vi "DataLogViewer.vi"() -> ()   [LabVIEW 2017]
uses:
  <vilib>/Utility/miscctls.llb/LVRowAndColumnTypeDef.ctl
  <vilib>/Utility/miscctls.llb/LVRowAndColumnUnsignedTypeDef.ctl
  <vilib>/Utility/sysdir.llb/System Directory Type.ctl
  <vilib>/Utility/NIReport.llb/Append Image to Report (path wrap).vi
  <vilib>/Utility/file.llb/Read Delimited Spreadsheet (string).vi
  <vilib>/Utility/NIReport.llb/NI_report.lvclass
  <vilib>/Utility/NIReport.llb/NI_ReportGenerationCore.lvlib
panel:
  in  "Print":bool
  in  "Explorer":bool
  out "SearchOut":T1
  in  "Search":bool
  in  "STR_Search":string caption="Search..."
  in  "Down":bool
  in  "Top":bool
  out "ResultGraph":string[](array[string])
  out "ResultTest":string[][](array[string])
  in  "Tab Control":enum32{"RESULT", "GRAPH"}(tab)
  out "PRODUCT No.":string
  out "LANE  No.":string
  out "LASER  No.":string
  out "RESULT":string
  out "QR Code":string
  out "Vision Pin":string
  out "Vision Pad":string
  out "LIN WDW Lock":string
  out "LIN AS Auto":string
  out "LIN AS Down":string
  out "LIN AS Up":string
  out "LIN DR Auto":string
  out "LIN DR Down":string
  out "LIN DR Up":string
  out "RL Man Down":string
  out "RL Man Up":string
  out "FL Auto Down":string
  out "FL Auto Up":string
  out "FL Man Down":string
  out "FL Man Up":string
  out "RR Man Down":string
  out "RR Man Up":string
  out "FR Auto Down":string
  out "FR Auto Up":string
  out "FR Man Down":string
  out "FR Man Up":string
  out "Door Unlocked":string
  out "Door Lock":string
  out "WDW Unlocked":string
  out "WDW Locked":string
  out "Megga Test":string
  out "RLG_Up":picture
  out "RLG_Down":picture
  out "FLG_Up":picture
  out "FLG_Down":picture
  out "RRG_Up":picture
  out "RRG_Down":picture
  out "FRG_Up":picture
  out "FRG_Down":picture
  out "DLG_Unlock":picture
  out "DLG_Lock":picture
  out "WDWG_Unlock":picture
  out "WDWG_Lock":picture
  out "FileCount":string
  out "Display":bool
  in  "TableType":string(combo)="VIEW ALL"
  out "Folder Table":string[][](table)
  in  "RefreshFolderList":bool
  out "DataC4":string[](array[string])
  out "PathC3":path
  out "PathC2":path
  out "DataC3":string[](array[string])
  out "DataC2":string[](array[string])
  out "DataC1":string[](array[string])
  out "PathC1":path
  out "PosC3":T2
  out "PosC2":T2
  in  "MasterPath":path=path "D:/Output"
  out "PosC1":T2
  # "RL Down"
  # "RL Up"
  # "FL Down"
  # "FL Up"
  # "RR Down"
  # "RR Up"
  # "FR Down"
  # "FR Up"
  # "Door Lock"
  # "Door Unlock"
  # "WDW Lock"
  # "WDW Unlock"
  # "DATA LOGGER"
  # "DATA LOGGER"
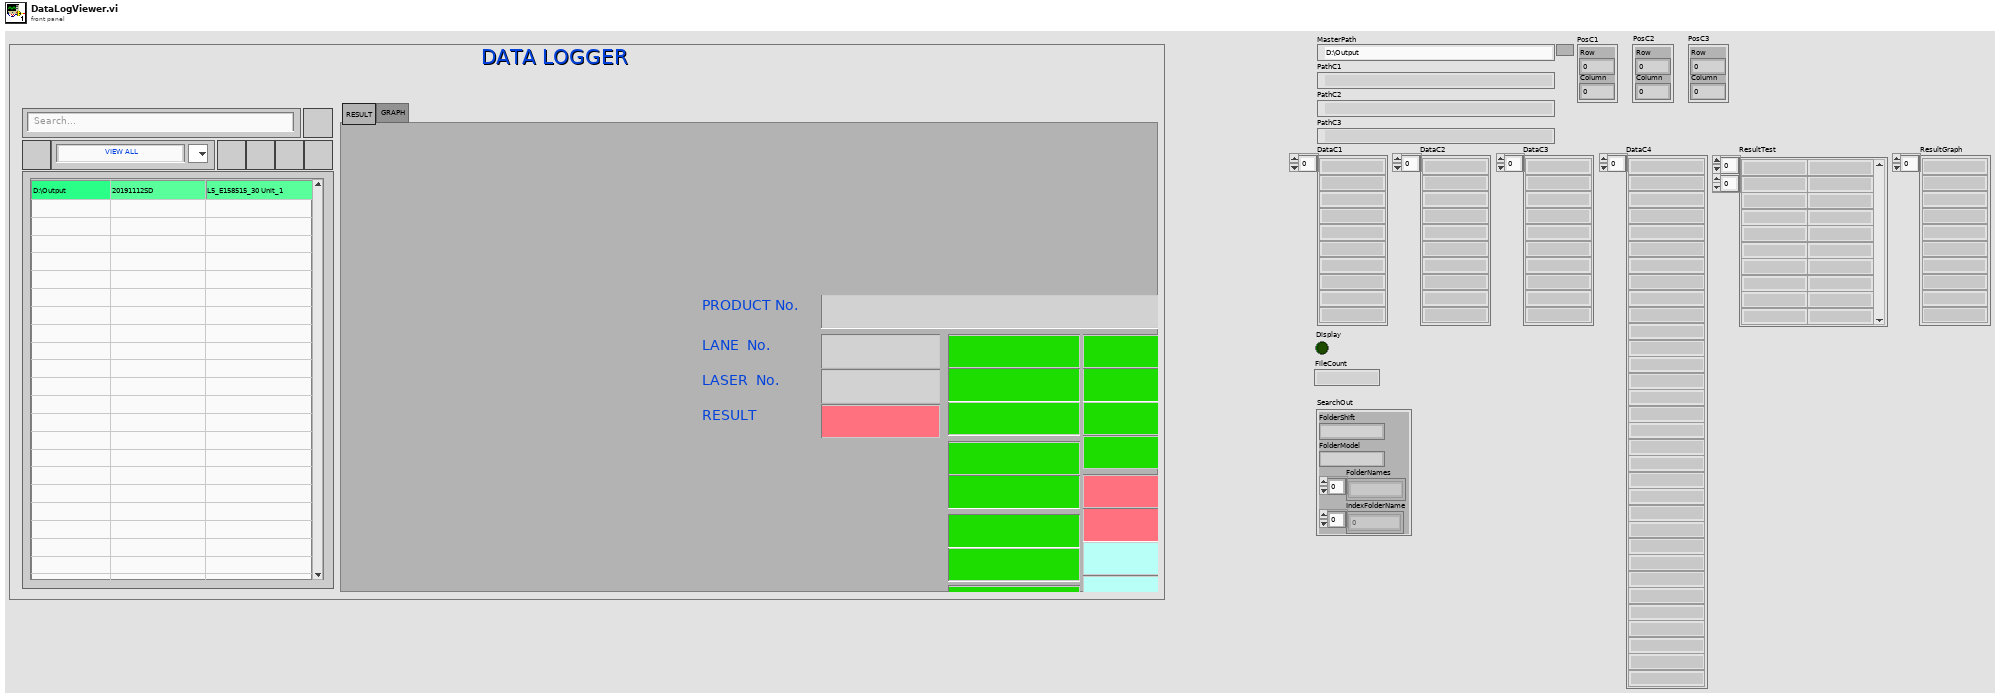
[diagram p1: front panel]
types:
  T1 = cluster{"FolderShift":string, "FolderModel":string, "FolderNames":string[], "IndexFolderName":i32[]}
  T2 = typedef "LVRowAndColumnTypeDef.ctl" = cluster{"Row":i32, "Column":i32}
  T3 = typedef "LVRowAndColumnUnsignedTypeDef.ctl" = cluster{"Row":u32, "Column":u32}
  T4 = enum16{"Standard Report", "HTML", "Word", "Excel"}
  T5 = enum16{"maximized", "minimized", "normal", "no change"}
  T6 = cluster{"top":dbl, "left":dbl, "right":dbl, "bottom":dbl}
  T7 = typedef "System Directory Type.ctl" = i32
  T8 = typedef "imagedata.ctl" = cluster{"image type":i32, "image depth":i32, "image":u8[], "mask":u8[], "colors":u32[], "Rectangle":cluster{"left":i16, "top":i16, "right":i16, "bottom":i16}}
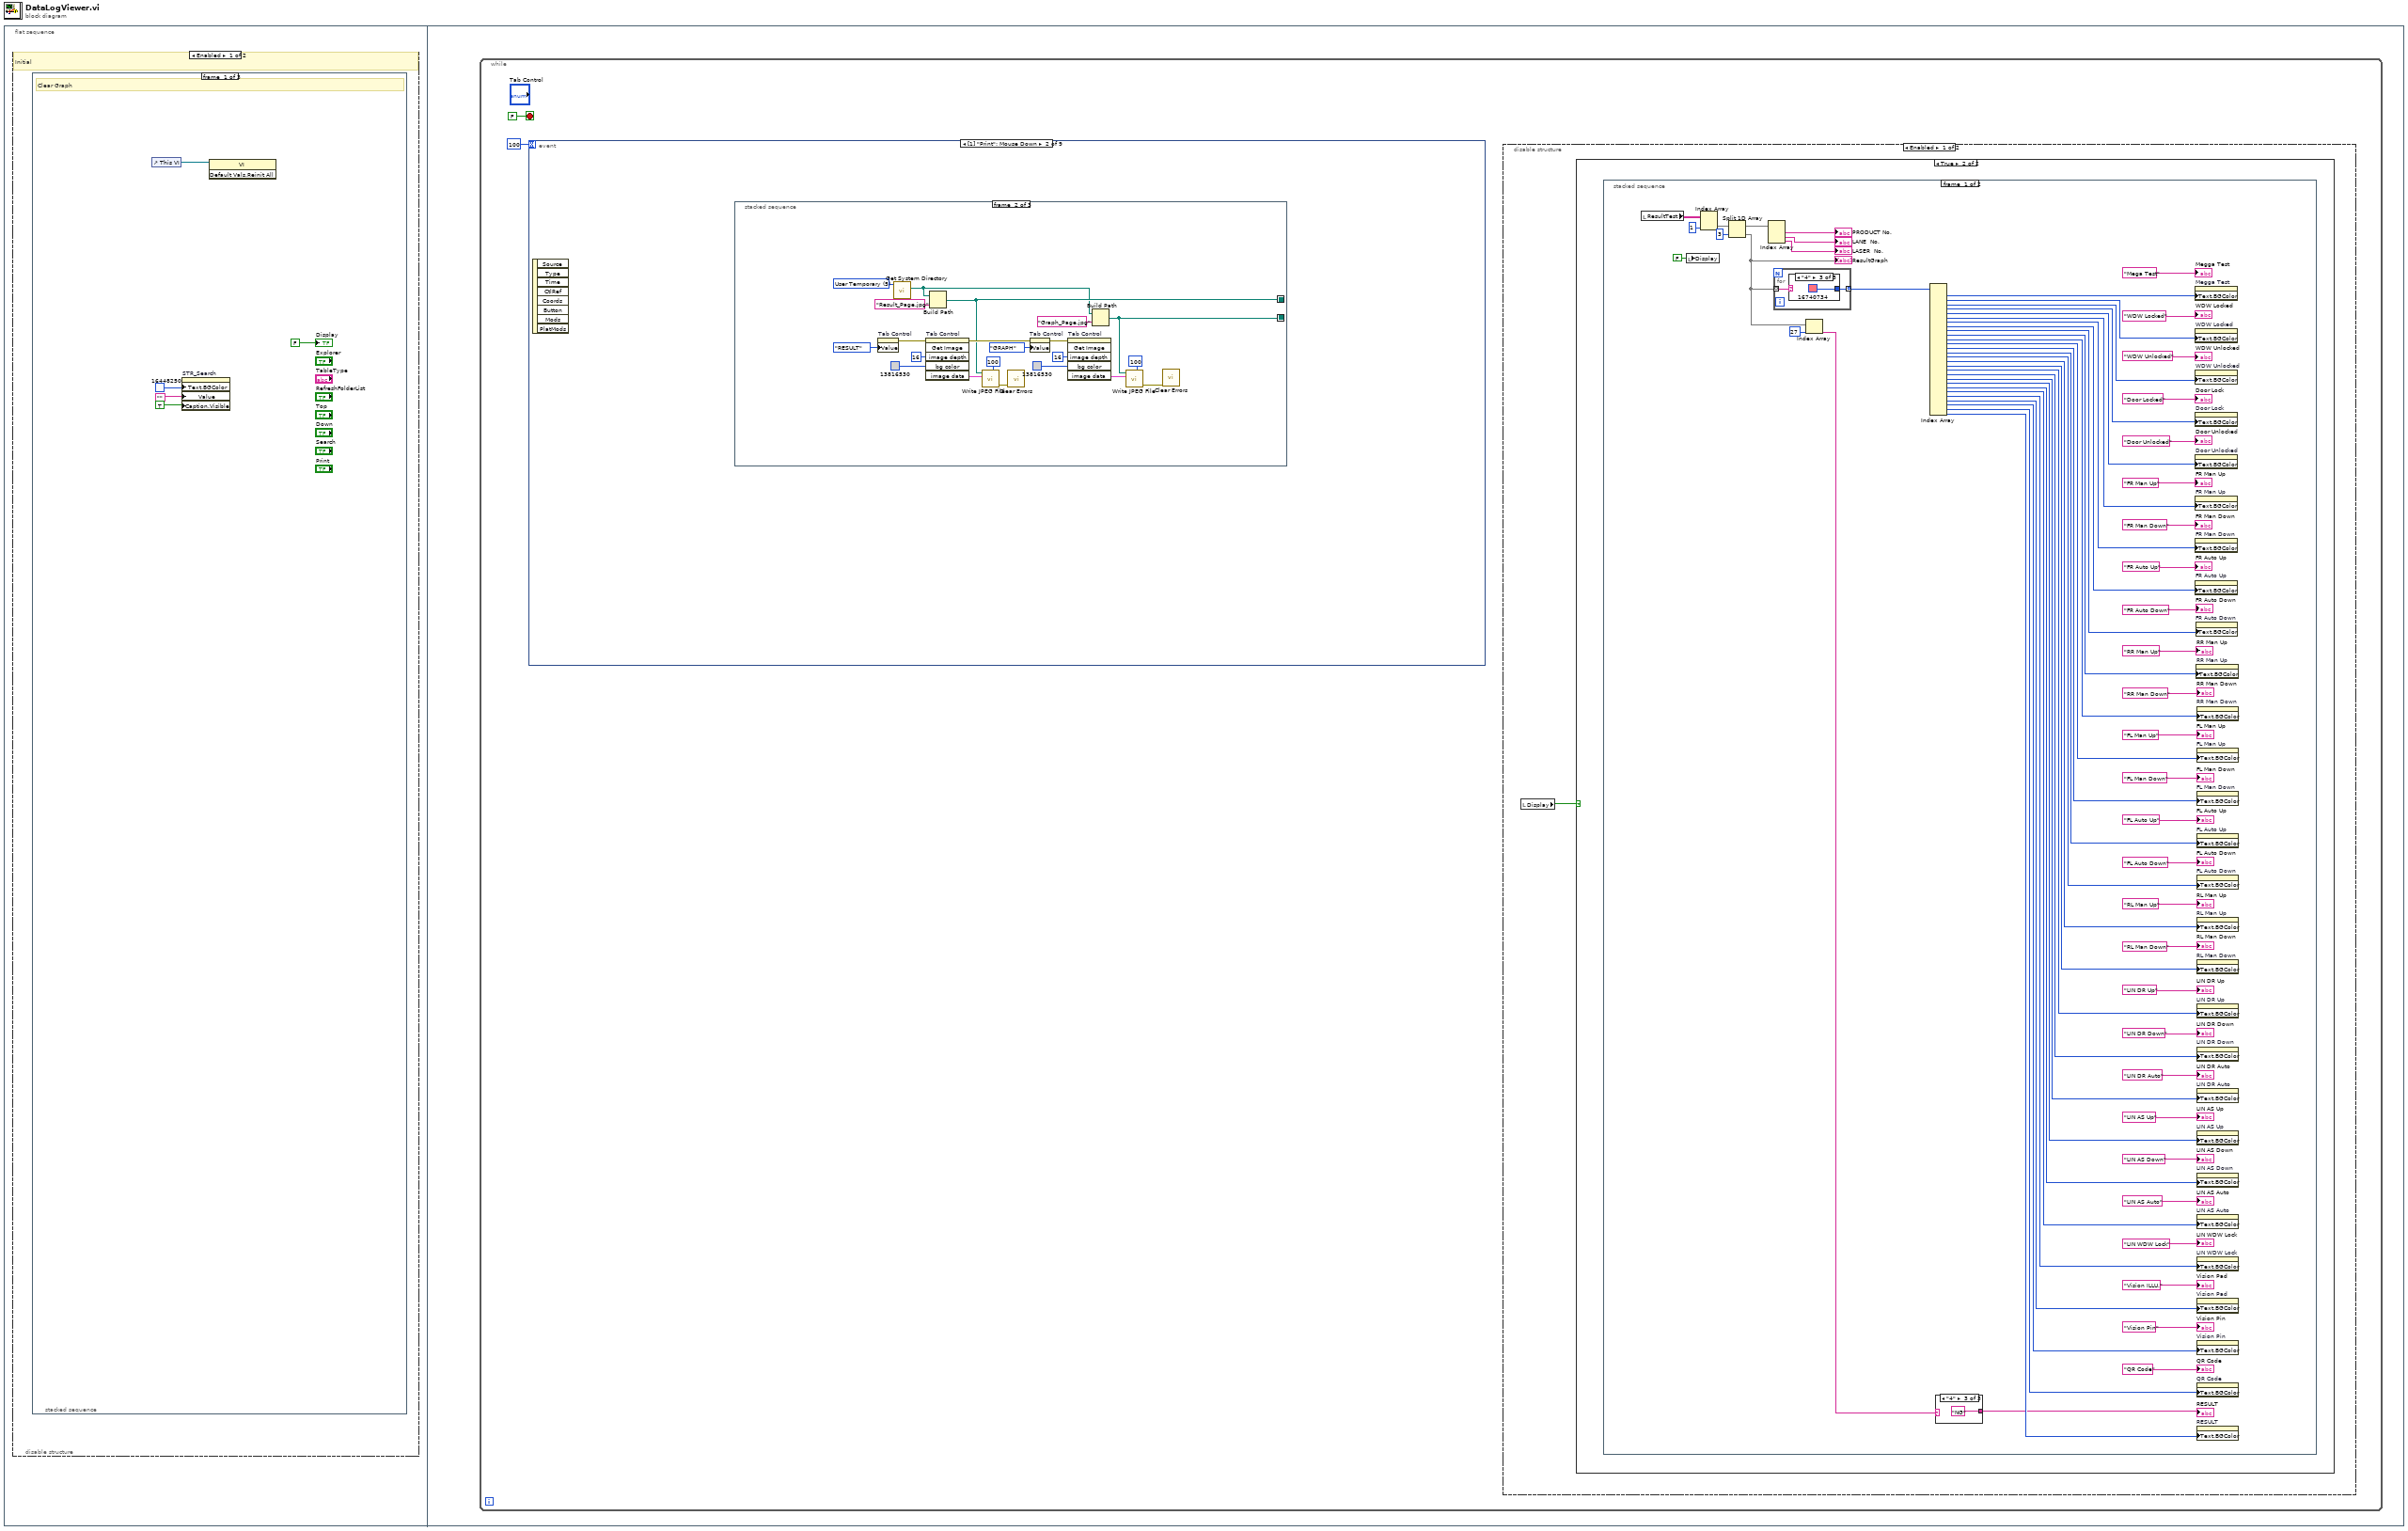
[diagram p0: block diagram]
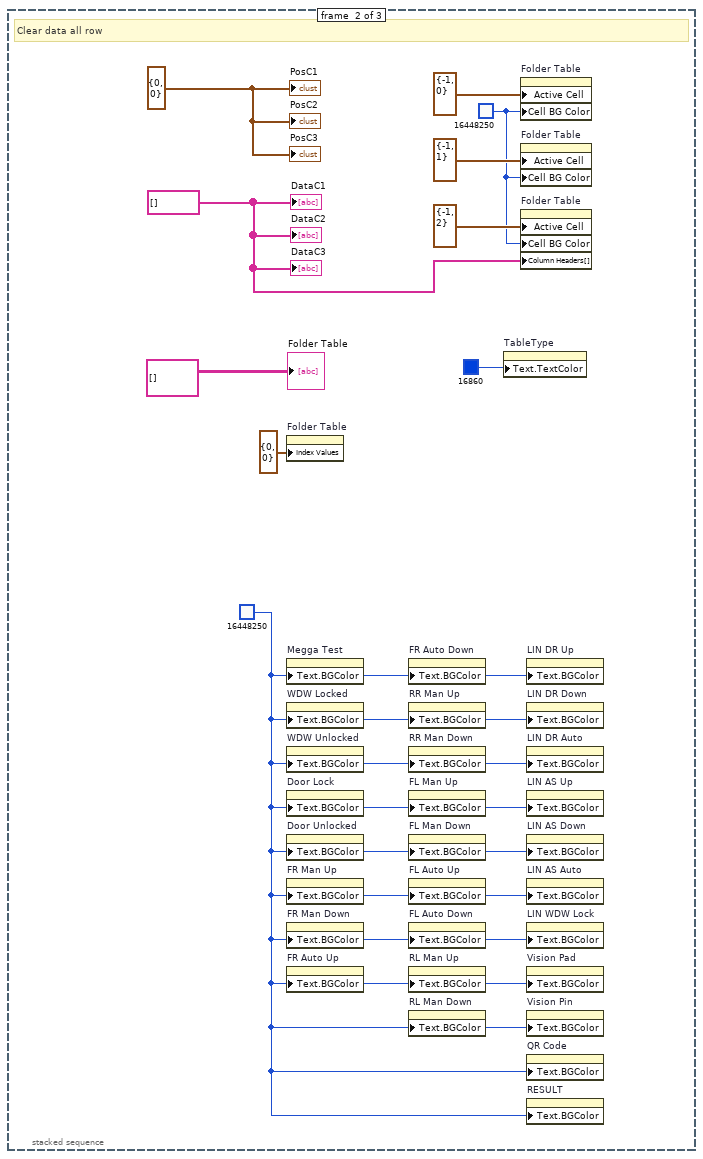
[diagram p2: hidden frame]
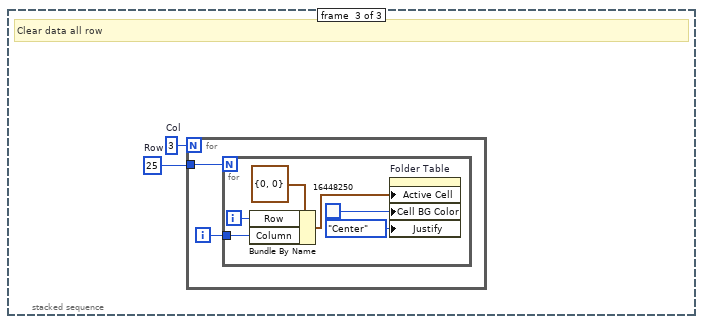
[diagram p3: hidden frame]
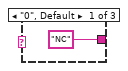
[diagram p6: hidden frame]
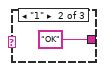
[diagram p7: hidden frame]
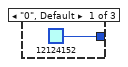
[diagram p8: hidden frame]
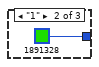
[diagram p9: hidden frame]
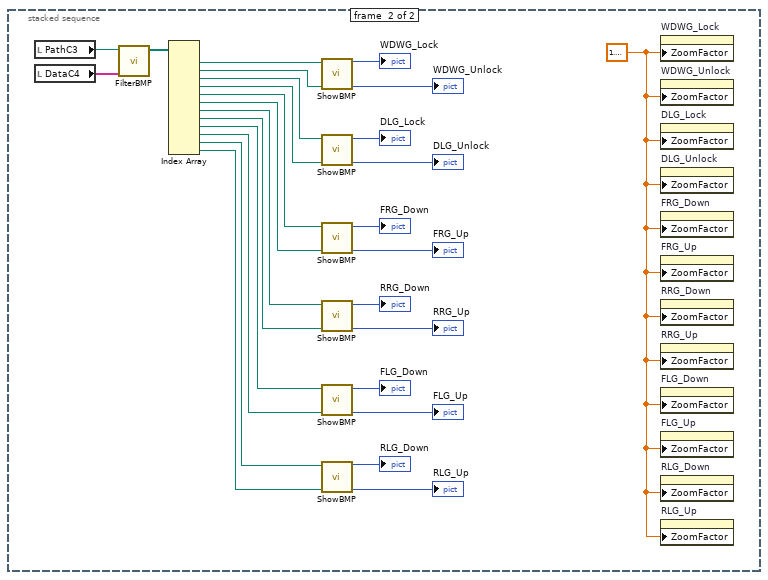
[diagram p10: hidden frame]
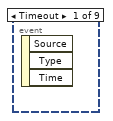
[diagram p12: hidden frame]
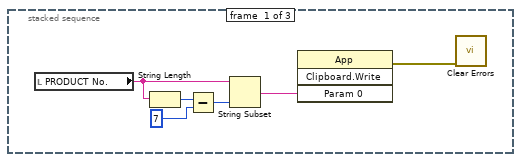
[diagram p13: hidden frame]
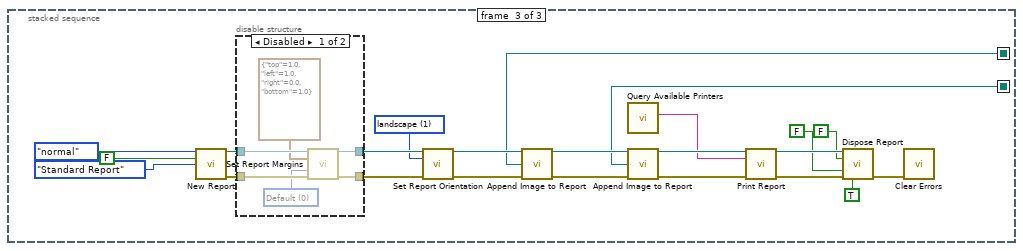
[diagram p14: hidden frame]
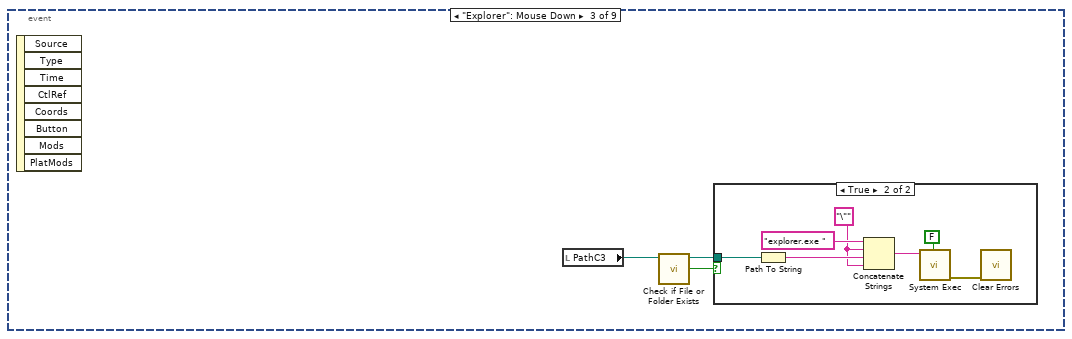
[diagram p16: hidden frame]
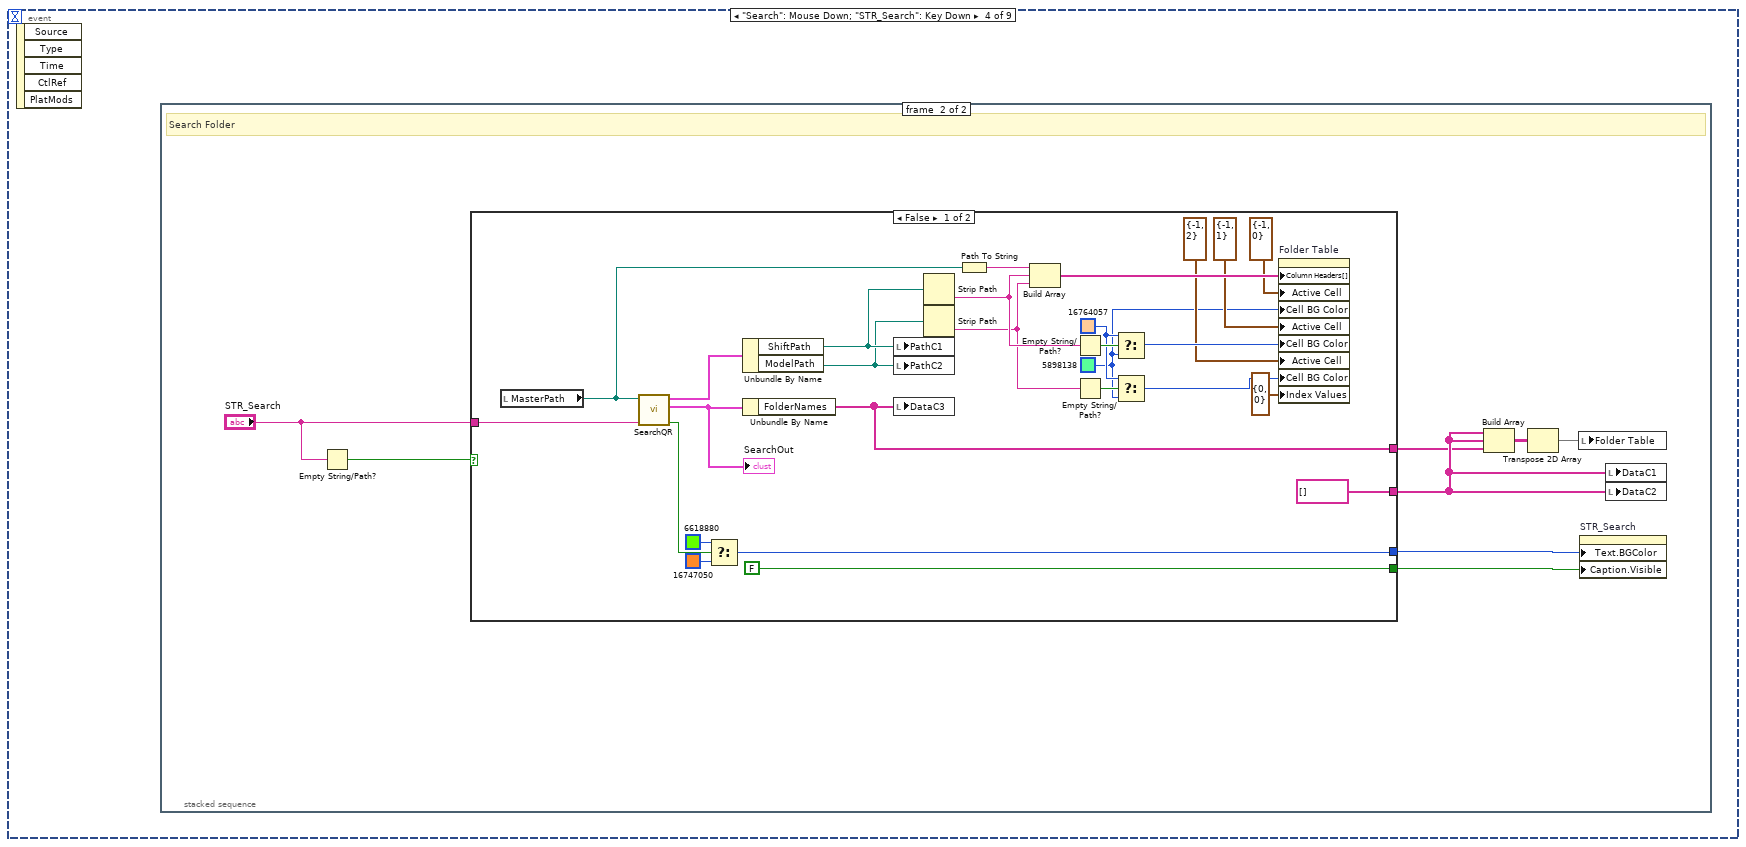
[diagram p18: hidden frame]
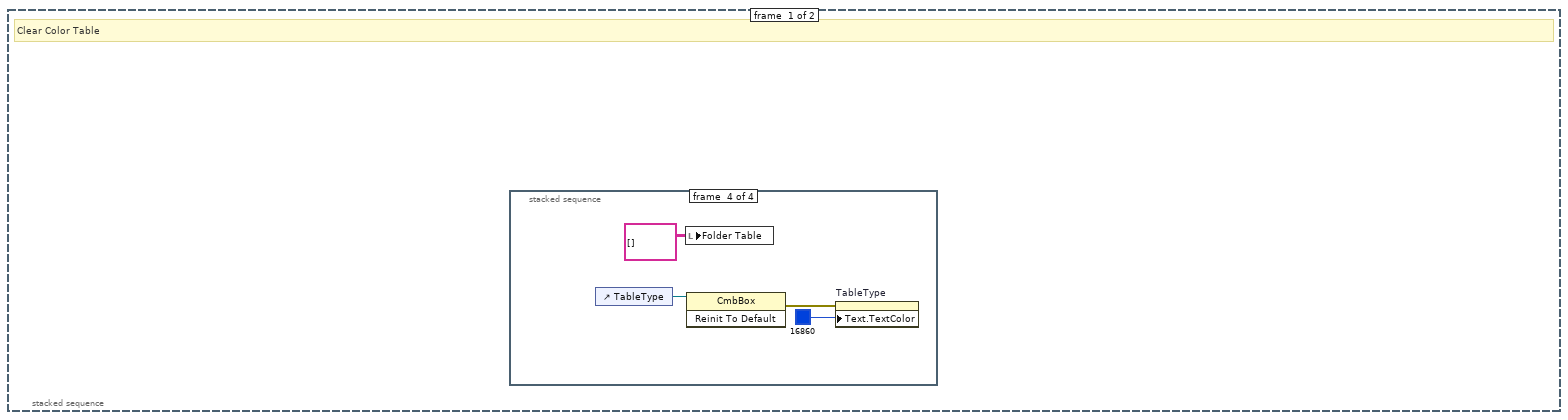
[diagram p19: hidden frame]
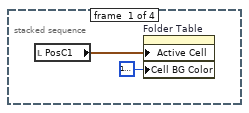
[diagram p20: hidden frame]
diagram:
  n1 = flat-sequence {
    frame #0 {
      n2 = disable-structure shown="Enabled" {
        frame Enabled {
          # "Initial"
          n3 = stacked-sequence {
            frame #0 {
              # "Clear Graph"
              n4 = control-ref of="This VI"() -> (w5:refnum<vi>)
              n5 = property on="STR_Search" class="Str"("Text.BGColor"=u32 16448250, "Value"="", "Caption.Visible"=TRUE) -> ()  [unwired: 2 in, 2 out]
              n6 = invoke class="VI" method="Default Vals.Reinit All"(reference=w5) -> ()  [unwired: 2 in, 3 out]
              "Display" <- FALSE ("Display")
            }
            frame #1 {
              w7 = u32 16448250
              w10 = u32 16448250
              w9 = string[] [] ("DataC1")
              w14 = T2 {"Row"=0, "Column"=0} ("LastPositionTable")
              # "Clear data all row"
              n7 = property on="Folder Table" class="Tbl (strict)"("Index Values"=T3 {"Row"=0, "Column"=0}) -> ()  [unwired: 2 in, 2 out]
              n8 = property on="Megga Test" class="Str"("Text.BGColor"=w7) -> ()  [unwired: 2 in, 2 out]
              n9 = property on="WDW Locked" class="Str"("Text.BGColor"=w7) -> ()  [unwired: 2 in, 2 out]
              n10 = property on="WDW Unlocked" class="Str"("Text.BGColor"=w7) -> ()  [unwired: 2 in, 2 out]
              n11 = property on="Door Lock" class="Str"("Text.BGColor"=w7) -> ()  [unwired: 2 in, 2 out]
              n12 = property on="Door Unlocked" class="Str"("Text.BGColor"=w7) -> ()  [unwired: 2 in, 2 out]
              n13 = property on="FR Man Up" class="Str"("Text.BGColor"=w7) -> ()  [unwired: 2 in, 2 out]
              n14 = property on="FR Man Down" class="Str"("Text.BGColor"=w7) -> ()  [unwired: 2 in, 2 out]
              n15 = property on="FR Auto Up" class="Str"("Text.BGColor"=w7) -> ()  [unwired: 2 in, 2 out]
              n16 = property on="FR Auto Down" class="Str"("Text.BGColor"=w7) -> ()  [unwired: 2 in, 2 out]
              n17 = property on="RR Man Up" class="Str"("Text.BGColor"=w7) -> ()  [unwired: 2 in, 2 out]
              n18 = property on="RR Man Down" class="Str"("Text.BGColor"=w7) -> ()  [unwired: 2 in, 2 out]
              n19 = property on="FL Man Up" class="Str"("Text.BGColor"=w7) -> ()  [unwired: 2 in, 2 out]
              n20 = property on="FL Man Down" class="Str"("Text.BGColor"=w7) -> ()  [unwired: 2 in, 2 out]
              n21 = property on="FL Auto Up" class="Str"("Text.BGColor"=w7) -> ()  [unwired: 2 in, 2 out]
              n22 = property on="FL Auto Down" class="Str"("Text.BGColor"=w7) -> ()  [unwired: 2 in, 2 out]
              n23 = property on="RL Man Up" class="Str"("Text.BGColor"=w7) -> ()  [unwired: 2 in, 2 out]
              n24 = property on="RL Man Down" class="Str"("Text.BGColor"=w7) -> ()  [unwired: 2 in, 2 out]
              n25 = property on="TableType" class="CmbBox"("Text.TextColor"=u32 16860) -> ()  [unwired: 2 in, 2 out]
              n26 = property on="Folder Table" class="Tbl (strict)"("Active Cell"=T2 {"Row"=-1, "Column"=0} ("Active Cell:Active Cell"), "Cell BG Color"=w10) -> ()  [unwired: 2 in, 2 out]
              n27 = property on="Folder Table" class="Tbl (strict)"("Active Cell"=T2 {"Row"=-1, "Column"=1} ("Active Cell:Active Cell"), "Cell BG Color"=w10) -> ()  [unwired: 2 in, 2 out]
              n28 = property on="Folder Table" class="Tbl (strict)"("Active Cell"=T2 {"Row"=-1, "Column"=2} ("Active Cell:Active Cell"), "Cell BG Color"=w10, "Column Headers[]"=w9) -> ()  [unwired: 2 in, 2 out]
              n29 = property on="LIN DR Up" class="Str"("Text.BGColor"=w7) -> ()  [unwired: 2 in, 2 out]
              n30 = property on="LIN DR Down" class="Str"("Text.BGColor"=w7) -> ()  [unwired: 2 in, 2 out]
              n31 = property on="LIN DR Auto" class="Str"("Text.BGColor"=w7) -> ()  [unwired: 2 in, 2 out]
              n32 = property on="LIN AS Up" class="Str"("Text.BGColor"=w7) -> ()  [unwired: 2 in, 2 out]
              n33 = property on="LIN AS Down" class="Str"("Text.BGColor"=w7) -> ()  [unwired: 2 in, 2 out]
              n34 = property on="LIN AS Auto" class="Str"("Text.BGColor"=w7) -> ()  [unwired: 2 in, 2 out]
              n35 = property on="LIN WDW Lock" class="Str"("Text.BGColor"=w7) -> ()  [unwired: 2 in, 2 out]
              n36 = property on="Vision Pad" class="Str"("Text.BGColor"=w7) -> ()  [unwired: 2 in, 2 out]
              n37 = property on="Vision Pin" class="Str"("Text.BGColor"=w7) -> ()  [unwired: 2 in, 2 out]
              n38 = property on="QR Code" class="Str"("Text.BGColor"=w7) -> ()  [unwired: 2 in, 2 out]
              n39 = property on="RESULT" class="Str"("Text.BGColor"=w7) -> ()  [unwired: 2 in, 2 out]
              "Folder Table" <- string[][] [] ("Folder Table")
              "PosC1" <- w14
              "PosC2" <- w14
              "PosC3" <- w14
              "DataC1" <- w9
              "DataC2" <- w9
              "DataC3" <- w9
            }
            frame #2 {
              w16 = u32 25  # Row
              w17 = 3  # Col
              # "Clear data all row"
              n40 = for {
                N: w17 -> [_]
                tunnel: w16 -> [w19]
                i -> [w18]
                n41 = for {
                  N: w19 -> [_]
                  tunnel: w18 -> [w21]
                  i -> [w22]
                  n42 = Bundle By Name(cluster=T2 {"Row"=0, "Column"=0} ("Active Cell:Active Cell"), "Row"=w22, "Column"=w21) -> (w23:T2)
                  n43 = property on="Folder Table" class="Tbl (strict)"("Active Cell"=w23, "Cell BG Color"=u32 16448250, "Justify"=enum16{"Left", "Center", "Right"}."Center" ("Active Cell:Cell Justification")) -> ()  [unwired: 2 in, 2 out]
                }
              }
            }
          }
        }
        frame Disabled {
        }
      }
    }
    frame #1 {
      n44 = while {
        stop <- FALSE stop-if-true
        n45 = event shown="[1] \"Print\": Mouse Down" {
          selector: _ -> [_ _ _ _ _ _ _ _ _]
          dyn-events: _ -> [_ _ _ _ _ _ _ _ _]
          timeout: 100 -> [_ _ _ _ _ _ _ _ _]
          event Timeout {
            n46 = event-data() -> ()  [unwired: 1 in, 3 out]
          }
          event "Print": Mouse Down {
            n47 = event-data() -> ()  [unwired: 1 in, 8 out]
            n48 = stacked-sequence {
              seq-local: [_ w145 _] -> [_ _ w164]
              seq-local: [_ w143 _] -> [_ _ w163]
              frame #0 {
                n49 = local read "PRODUCT No."() -> (w139:string)
                n50 = String Length(string=w139) -> (length=w138:i32)
                n51 = Subtract(x=w138, y=7) -> (x-y=w136:i32)
                n52 = String Subset(string=w139, length (rest)=w136) -> (substring=w135:string)  [unwired: 1 in]
                n53 = invoke class="App" method="Clipboard.Write"("Param 0"=w135) -> (error out=w134:errorcluster)  [unwired: 3 in, 3 out]
                n54 = call <vilib>:"Clear Errors.vi"("error in (no error)"=w134) -> ()  [unwired: 5 in, 2 out]
              }
              frame #1 {
                w147 = T7 5 items=["User Home"=0, "User Desktop"=1, "User Documents"=2, "User Application Data"=3, "User Preferences"=4, "User Temporary"=5, "Public Documents"=6, "Public Application Data"=7, "Public Preferences"=8, "Public Cache"=13, "System Core Libraries"=9, "System Installed Libraries"=10, "Application Files"=11, "Boot Volume Root"=12] ("system directory type")
                n55 = property on="Tab Control" class="TabCtl (strict)"("Value"=enum32{"RESULT", "GRAPH"}."RESULT" ("Tab Control")) -> (error out=w156:errorcluster)  [unwired: 2 in, 1 out]
                n56 = call <vilib>:"Get System Directory.vi"("system directory type"=w147) -> ("system directory"=w142:path)  [unwired: 10 in]
                n57 = invoke on="Tab Control" class="TabCtl (strict)" method="Get Image"(error in=w156, "image depth"=16 ("Image Depth"), "bg color"=u32 13816530) -> (error out=w153:errorcluster, "image data"=w158:T8)  [unwired: 3 in, 4 out]
                n58 = Build Path(base path=w142, name or relative path="Result_Page.jpg") -> (appended path=w145:path)
                n59 = call <vilib>:"Write JPEG File.vi"("quality (80)"=100, "image data"=w158, "path to JPEG file"=w145) -> ("error out"=w140:errorcluster)  [unwired: 7 in, 1 out]
                n60 = call <vilib>:"Clear Errors.vi"("error in (no error)"=w140) -> ()  [unwired: 5 in, 2 out]
                n61 = property on="Tab Control" class="TabCtl (strict)"(error in=w153, "Value"=enum32{"RESULT", "GRAPH"}."GRAPH" ("Tab Control")) -> (error out=w148:errorcluster)  [unwired: 1 in, 1 out]
                n62 = invoke on="Tab Control" class="TabCtl (strict)" method="Get Image"(error in=w148, "image depth"=16 ("Image Depth"), "bg color"=u32 13816530) -> ("image data"=w151:T8)  [unwired: 3 in, 5 out]
                n63 = Build Path(base path=w142, name or relative path="Graph_Page.jpg") -> (appended path=w143:path)
                n64 = call <vilib>:"Write JPEG File.vi"("quality (80)"=100, "image data"=w151, "path to JPEG file"=w143) -> ("error out"=w141:errorcluster)  [unwired: 7 in, 1 out]
                n65 = call <vilib>:"Clear Errors.vi"("error in (no error)"=w141) -> ()  [unwired: 5 in, 2 out]
              }
              frame #2 {
                w168 = 1 items=["portrait", "landscape"] ("orientation (portrait)")
                n66 = call <vilib>:"New Report.vi"("window state (normal)"=T5."normal", "display alerts? (F)"=FALSE, "report type"=T4."Standard Report") -> ("report out"=w175:refnum<class "NI_report.lvclass">, "error out"=w174:errorcluster)  [unwired: 11 in]
                n67 = disable-structure shown="Disabled" {
                  disable-tunnel: w175 -> [w189 w191]
                  disable-tunnel: w174 -> [w188 w190]
                  disable-tunnel: [w187 w190] -> w173
                  disable-tunnel: [w186 w191] -> w172
                  frame Disabled {
                    w184 = u16 0 items=["Default", "US", "Metric"] ("measurement system (default)")
                    n68 = call-dynamic "Set Report Margins.vi"("report in"=w189, "margins (1.00)"=T6 {"top"=1.0, "left"=1.0, "right"=0.0, "bottom"=1.0}, "measurement system (default)"=w184, "error in (no error)"=w188) -> ("report out"=w186:refnum<class "NI_report.lvclass">, "error out"=w187:errorcluster)  [unwired: 9 in, 1 out]
                  }
                  frame Enabled {
                  }
                }
                n69 = call-dynamic "Set Report Orientation.vi"("report in"=w172, "orientation (portrait)"=w168, "error in (no error)"=w173) -> ("report out"=w178:refnum<class "NI_report.lvclass">, "error out"=w179:errorcluster)  [unwired: 11 in]
                n70 = call-poly <vilib>:"Append Image to Report.vi"("report in"=w178, "path or URL of image"=w164, "error in (no error)"=w179) -> ("report out"=w180:refnum<class "NI_report.lvclass">, "error out"=w181:errorcluster)  [unwired: 9 in, 2 out]
                n71 = call <vilib>:"Query Available Printers.vi"() -> ("default printer"=w162:string)  [unwired: 9 in, 2 out]
                n72 = call-poly <vilib>:"Append Image to Report.vi"("report in"=w180, "path or URL of image"=w163, "error in (no error)"=w181) -> ("report out"=w182:refnum<class "NI_report.lvclass">, "error out"=w183:errorcluster)  [unwired: 9 in, 2 out]
                n73 = call-dynamic "Print Report.vi"("report in"=w182, "printer name (default)"=w162, "error in (no error)"=w183) -> ("report out"=w176:refnum<class "NI_report.lvclass">, "error out"=w177:errorcluster)  [unwired: 11 in]
                n74 = call-dynamic "Dispose Report.vi"("report in"=w176, "wait until printing completed? (T)"=FALSE, "save changes? (F)"=FALSE, "error in (no error)"=w177, "close report? (T)"=TRUE) -> ("error out"=w161:errorcluster)  [unwired: 10 in]
                n75 = call <vilib>:"Clear Errors.vi"("error in (no error)"=w161) -> ()  [unwired: 5 in, 2 out]
              }
            }
          }
          event "Explorer": Mouse Down {
            n76 = event-data() -> ()  [unwired: 1 in, 8 out]
            n77 = local read "PathC3"() -> (w192:path)
            n78 = call <vilib>:"Check if File or Folder Exists.vi"("path"=w192) -> ("file or folder exists?"=w193:bool, "dup path"=w194:path)  [unwired: 8 in, 1 out]
            n79 = case shown="True" w193 {
              tunnel: w194 -> [_ w198]
              frame False {
              }
              frame True {
                w195 = "\"" ("string")
                n80 = Path To String(path=w198) -> (string=w196:string)
                n81 = Concatenate Strings("explorer.exe " ("string"), w195, w196, w195) -> (w199:string)
                n82 = call <vilib>:"System Exec.vi"("wait until completion? (T)"=FALSE, "command line"=w199) -> ("error out"=w197:errorcluster)  [unwired: 6 in, 3 out]
                n83 = call <vilib>:"Clear Errors.vi"("error in (no error)"=w197) -> ()  [unwired: 5 in, 2 out]
              }
            }
          }
          event "Search": Mouse Down; "STR_Search": Key Down {
            n84 = event-data() -> ()  [unwired: 1 in, 5 out]
            n85 = stacked-sequence {
              frame #0 {
                # "Clear Color Table"
                n86 = stacked-sequence {
                  frame #0 {
                    n87 = local read "PosC1"() -> (w202:T2)
                    n88 = property on="Folder Table" class="Tbl (strict)"("Active Cell"=w202, "Cell BG Color"=u32 16777225) -> ()  [unwired: 2 in, 2 out]
                  }
                  frame #1 {
                    n89 = local read "PosC2"() -> (w204:T2)
                    n90 = property on="Folder Table" class="Tbl (strict)"("Active Cell"=w204, "Cell BG Color"=u32 16777225) -> ()  [unwired: 2 in, 2 out]
                  }
                  frame #2 {
                    n91 = local read "PosC3"() -> (w206:T2)
                    n92 = property on="Folder Table" class="Tbl (strict)"("Active Cell"=w206, "Cell BG Color"=u32 16777225) -> ()  [unwired: 2 in, 2 out]
                  }
                  frame #3 {
                    n93 = control-ref of="TableType"() -> (w209:refnum<vi>)
                    n94 = local write "Folder Table"(string[][] [] ("Folder Table")) -> ()
                    n95 = invoke class="CmbBox" method="Reinit To Default"(reference=w209) -> (error out=w210:errorcluster)  [unwired: 2 in, 2 out]
                    n96 = property on="TableType" class="CmbBox"(error in=w210, "Text.TextColor"=u32 16860) -> ()  [unwired: 1 in, 2 out]
                  }
                }
              }
              frame #1 {
                # "Search Folder"
                n97 = Empty String/Path?(string/path="STR_Search") -> (empty?=w218:bool)
                n98 = case shown="False" w218 {
                  tunnel: "STR_Search" -> [w246 _]
                  tunnel: [string[] [] ("element") w249] -> w215
                  tunnel: [w222 w249] -> w214
                  tunnel: [FALSE ("Caption.Visible") TRUE ("Caption.Visible")] -> w213
                  tunnel: [w221 u32 16448250] -> w212
                  frame False {
                    w232 = u32 16764057
                    w227 = u32 5898138
                    n99 = local read "MasterPath"() -> (w238:path)
                    n100 = call "SearchQR.vi"("QR_Code"=w246, "MasterPath"=w238) -> ("FolderOK"=w243:bool, "Folder"=w242:T1, "Path"=w241:cluster{"ShiftPath":path, "ModelPath":path})  [unwired: 7 in]
                    "SearchOut" <- w242
                    n101 = Select(t=u32 6618880, s=w243, f=u32 16747050) -> (s? t:f=w221:u32)
                    n102 = Unbundle By Name(w241) -> ("ShiftPath"=w237:path, "ModelPath"=w236:path)
                    n103 = Unbundle By Name(w242) -> ("FolderNames"=w222:string[])
                    n104 = local write "PathC1"(w237) -> ()
                    n105 = local write "PathC2"(w236) -> ()
                    n106 = local write "DataC3"(w222) -> ()
                    n107 = Strip Path(path=w237) -> (name=w226:string)  [unwired: 1 out]
                    n108 = Strip Path(path=w236) -> (name=w225:string)  [unwired: 1 out]
                    n109 = Path To String(path=w238) -> (string=w239:string)
                    n110 = Build Array(w239, w226, w225) -> (w240:string[])
                    n111 = Empty String/Path?(string/path=w226) -> (empty?=w233:bool)
                    n112 = Empty String/Path?(string/path=w225) -> (empty?=w234:bool)
                    n113 = Select(t=w232, s=w233, f=w227) -> (s? t:f=w231:u32)
                    n114 = Select(t=w232, s=w234, f=w227) -> (s? t:f=w230:u32)
                    n115 = property on="Folder Table" class="Tbl (strict)"("Column Headers[]"=w240, "Active Cell"=T2 {"Row"=-1, "Column"=0} ("Active Cell:Active Cell"), "Cell BG Color"=w227, "Active Cell"=T2 {"Row"=-1, "Column"=1} ("Active Cell:Active Cell"), "Cell BG Color"=w231, "Active Cell"=T2 {"Row"=-1, "Column"=2} ("Active Cell:Active Cell"), "Cell BG Color"=w230, "Index Values"=T3 {"Row"=0, "Column"=0}) -> ()  [unwired: 2 in, 2 out]
                  }
                  frame True {
                    w249 = string[] [] ("FolderNames")
                  }
                }
                n116 = Build Array(w215, w215, w214) -> (w217:string[][])
                n117 = Transpose 2D Array(2D array=w217) -> (transposed array=w216:string[][])
                n118 = local write "Folder Table"(w216) -> ()
                n119 = property on="STR_Search" class="Str"("Text.BGColor"=w212, "Caption.Visible"=w213) -> ()  [unwired: 2 in, 2 out]
                n120 = local write "DataC1"(w215) -> ()
                n121 = local write "DataC2"(w215) -> ()
              }
            }
          }
          event "Top": Mouse Down {
            n122 = event-data() -> ()  [unwired: 1 in, 8 out]
            n123 = property on="Folder Table" class="Tbl (strict)"("Index Values"=T3 {"Row"=0, "Column"=0}) -> ()  [unwired: 2 in, 2 out]
          }
          event "Down": Mouse Down {
            w253 = 22 ("y")
            n124 = event-data() -> ()  [unwired: 1 in, 8 out]
            n125 = local read "DataC1"() -> (w266:string[])
            n126 = local read "DataC2"() -> (w265:string[])
            n127 = local read "DataC3"() -> (w264:string[])
            n128 = Array Size(array=w266) -> (size(s)=w263:i32)
            n129 = Array Size(array=w265) -> (size(s)=w262:i32)
            n130 = Array Size(array=w264) -> (size(s)=w260:i32)
            n131 = Max & Min(x=w263, y=w262) -> (max(x,y)=w261:i32)  [unwired: 1 out]
            n132 = Max & Min(x=w261, y=w260) -> (max(x,y)=w254:i32)  [unwired: 1 out]
            n133 = Subtract(x=w254, y=w253) -> (x-y=w252:i32)
            n134 = Greater?(x=w254, y=w253) -> (0:w256:bool)
            n135 = Select(t=w252, s=w256, f=0 ("y")) -> (s? t:f=w251:i32)
            n136 = Bundle By Name(cluster=T3 {"Row"=0, "Column"=0} ("Index Values"), "Row"=w251, "Column"=u32 0) -> (w258:T3)
            n137 = property on="Folder Table" class="Tbl (strict)"("Index Values"=w258) -> ()  [unwired: 2 in, 2 out]
          }
          event "RefreshFolderList": Mouse Down {
            n138 = event-data() -> ()  [unwired: 1 in, 8 out]
            n139 = stacked-sequence {
              frame #0 {
                # "Clear color Table"
                n140 = stacked-sequence {
                  frame #0 {
                    n141 = local read "PosC1"() -> (w267:T2)
                    n142 = property on="Folder Table" class="Tbl (strict)"("Active Cell"=w267, "Cell BG Color"=u32 16777225) -> ()  [unwired: 2 in, 2 out]
                  }
                  frame #1 {
                    n143 = local read "PosC2"() -> (w269:T2)
                    n144 = property on="Folder Table" class="Tbl (strict)"("Active Cell"=w269, "Cell BG Color"=u32 16777225) -> ()  [unwired: 2 in, 2 out]
                  }
                  frame #2 {
                    n145 = local read "PosC3"() -> (w271:T2)
                    n146 = property on="Folder Table" class="Tbl (strict)"("Active Cell"=w271, "Cell BG Color"=u32 16777225) -> ()  [unwired: 2 in, 2 out]
                  }
                  frame #3 {
                    w273 = T2 {"Row"=0, "Column"=0} ("PosC1")
                    n147 = local write "PosC1"(w273) -> ()
                    n148 = local write "PosC2"(w273) -> ()
                    n149 = local write "PosC3"(w273) -> ()
                  }
                  frame #4 {
                    n150 = property on="STR_Search" class="Str"("Text.BGColor"=u32 16448250, "Value"="", "Caption.Visible"=TRUE) -> ()  [unwired: 2 in, 2 out]
                  }
                }
              }
              frame #1 {
                # "Clear data table"
                n151 = property on="Folder Table" class="Tbl (strict)"("Index Values"=T2 {"Row"=0, "Column"=0} ("Active Cell:Active Cell")) -> ()  [unwired: 2 in, 2 out]
                n152 = call <vilib>:"Check if File or Folder Exists.vi"("path"="MasterPath") -> ("file or folder exists?"=w280:bool, "dup path"=w279:path)  [unwired: 8 in, 1 out]
                n153 = case shown="True" w280 {
                  tunnel: w279 -> [_ w283]
                  frame False {
                  }
                  frame True {
                    w282 = enum16{"Left", "Center", "Right"}."Center" ("Active Cell:Cell Justification")
                    w281 = string[] [] ("element")
                    w291 = ""
                    n154 = Path To String(path=w283) -> (string=w292:string)
                    n155 = List Folder(path=w283) -> (folder names=w284:string[])  [unwired: 3 in, 3 out]
                    n156 = Build Array(w292, w291, w291) -> (w293:string[])
                    n157 = local write "DataC2"(w281) -> ()
                    n158 = local write "DataC3"(w281) -> ()
                    n159 = local write "DataC4"(w281) -> ()
                    n160 = property on="Folder Table" class="Tbl (strict)"("Column Headers[]"=w293) -> ()  [unwired: 2 in, 2 out]
                    n161 = property on="Folder Table" class="Tbl (strict)"("Active Cell"=T2 {"Row"=-1, "Column"=0} ("Active Cell:Active Cell"), "Cell BG Color"=u32 2817928, "Justify"=w282) -> ()  [unwired: 2 in, 2 out]
                    n162 = property on="Folder Table" class="Tbl (strict)"("Active Cell"=T2 {"Row"=-1, "Column"=1} ("Active Cell:Active Cell"), "Cell BG Color"=u32 16448250, "Justify"=w282) -> ()  [unwired: 2 in, 2 out]
                    n163 = property on="Folder Table" class="Tbl (strict)"("Active Cell"=T2 {"Row"=-1, "Column"=2} ("Active Cell:Active Cell"), "Cell BG Color"=u32 16448250, "Justify"=w282) -> ()  [unwired: 2 in, 2 out]
                    n164 = local write "DataC1"(w284) -> ()
                    n165 = Build Array(w284, w281, w281) -> (w295:string[][])
                    n166 = Transpose 2D Array(2D array=w295) -> (transposed array=w294:string[][])
                    n167 = local write "Folder Table"(w294) -> ()
                  }
                }
              }
              frame #2 {
                w296 = u32 16448250
                # "Clear background color"
                n168 = property on="Megga Test" class="Str"("Text.BGColor"=w296) -> ()  [unwired: 2 in, 2 out]
                n169 = property on="WDW Locked" class="Str"("Text.BGColor"=w296) -> ()  [unwired: 2 in, 2 out]
                n170 = property on="WDW Unlocked" class="Str"("Text.BGColor"=w296) -> ()  [unwired: 2 in, 2 out]
                n171 = property on="Door Lock" class="Str"("Text.BGColor"=w296) -> ()  [unwired: 2 in, 2 out]
                n172 = property on="Door Unlocked" class="Str"("Text.BGColor"=w296) -> ()  [unwired: 2 in, 2 out]
                n173 = property on="FR Man Up" class="Str"("Text.BGColor"=w296) -> ()  [unwired: 2 in, 2 out]
                n174 = property on="FR Man Down" class="Str"("Text.BGColor"=w296) -> ()  [unwired: 2 in, 2 out]
                n175 = property on="FR Auto Up" class="Str"("Text.BGColor"=w296) -> ()  [unwired: 2 in, 2 out]
                n176 = property on="FR Auto Down" class="Str"("Text.BGColor"=w296) -> ()  [unwired: 2 in, 2 out]
                n177 = property on="RR Man Up" class="Str"("Text.BGColor"=w296) -> ()  [unwired: 2 in, 2 out]
                n178 = property on="RR Man Down" class="Str"("Text.BGColor"=w296) -> ()  [unwired: 2 in, 2 out]
                n179 = property on="FL Man Up" class="Str"("Text.BGColor"=w296) -> ()  [unwired: 2 in, 2 out]
                n180 = property on="FL Man Down" class="Str"("Text.BGColor"=w296) -> ()  [unwired: 2 in, 2 out]
                n181 = property on="FL Auto Up" class="Str"("Text.BGColor"=w296) -> ()  [unwired: 2 in, 2 out]
                n182 = property on="FL Auto Down" class="Str"("Text.BGColor"=w296) -> ()  [unwired: 2 in, 2 out]
                n183 = property on="RL Man Up" class="Str"("Text.BGColor"=w296) -> ()  [unwired: 2 in, 2 out]
                n184 = property on="RL Man Down" class="Str"("Text.BGColor"=w296) -> ()  [unwired: 2 in, 2 out]
                n185 = property on="LIN DR Up" class="Str"("Text.BGColor"=w296) -> ()  [unwired: 2 in, 2 out]
                n186 = property on="LIN DR Down" class="Str"("Text.BGColor"=w296) -> ()  [unwired: 2 in, 2 out]
                n187 = property on="LIN DR Auto" class="Str"("Text.BGColor"=w296) -> ()  [unwired: 2 in, 2 out]
                n188 = property on="LIN AS Up" class="Str"("Text.BGColor"=w296) -> ()  [unwired: 2 in, 2 out]
                n189 = property on="LIN AS Down" class="Str"("Text.BGColor"=w296) -> ()  [unwired: 2 in, 2 out]
                n190 = property on="LIN AS Auto" class="Str"("Text.BGColor"=w296) -> ()  [unwired: 2 in, 2 out]
                n191 = property on="LIN WDW Lock" class="Str"("Text.BGColor"=w296) -> ()  [unwired: 2 in, 2 out]
                n192 = property on="Vision Pad" class="Str"("Text.BGColor"=w296) -> ()  [unwired: 2 in, 2 out]
                n193 = property on="Vision Pin" class="Str"("Text.BGColor"=w296) -> ()  [unwired: 2 in, 2 out]
                n194 = property on="QR Code" class="Str"("Text.BGColor"=w296) -> ()  [unwired: 2 in, 2 out]
                n195 = property on="RESULT" class="Str"("Text.BGColor"=w296) -> ()  [unwired: 2 in, 2 out]
              }
            }
          }
          event "Folder Table": Mouse Down {
            n196 = event-data() -> ()  [unwired: 1 in, 8 out]
            n197 = property on="Folder Table" class="Tbl (strict)"() -> ("EditPos"=w308:T2)  [unwired: 2 in, 2 out]
            n198 = Unbundle By Name(w308) -> ("Row"=w306:i32, "Column"=w302:i32)
            n199 = local read "STR_Search"() -> (w303:string)
            n200 = Empty String/Path?(string/path=w303) -> (empty?=w300:bool)
            n201 = Equal?(x=w302, y=2) -> (x = y?=w299:bool)
            n202 = Greater Or Equal To 0?(x=w306) -> (x >= 0?=w304:bool)
            n203 = Greater Or Equal To 0?(x=w302) -> (x >= 0?=w305:bool)
            n204 = Select(t=TRUE, s=w300, f=w299) -> (s? t:f=w297:bool)
            n205 = Compound Arithmetic op=AND(w304, w305, w297) -> (w307:bool)
            n206 = case shown="True" w307 {
              tunnel: w302 -> [_ w311]
              tunnel: w308 -> [_ w310]
              tunnel: w306 -> [_ w309]
              frame False {
              }
              frame True {
                n207 = case shown="0, Default" w311 {
                  tunnel: w310 -> [w319 w361 w451]
                  tunnel: w309 -> [w313 w355 w452]
                  frame 0, Default {
                    n208 = local read "MasterPath"() -> (w317:path)
                    n209 = local read "DataC1"() -> (w314:string[])
                    n210 = Index Array(array=w314, index=w313) -> (element=w318:string)
                    n211 = Build Path(base path=w317, name or relative path=w318) -> (appended path=w316:path)
                    "PathC1" <- w316
                    n212 = call <vilib>:"Check if File or Folder Exists.vi"("path"=w316) -> ("file or folder exists?"=w312:bool, "dup path"=w315:path)  [unwired: 8 in, 1 out]
                    n213 = case shown="True" w312 {
                      tunnel: w315 -> [_ w343]
                      frame False {
                      }
                      frame True {
                        w337 = string[] [] ("element")
                        n214 = List Folder(path=w343) -> (path out=w327:path, folder names=w320:string[])  [unwired: 3 in, 2 out]
                        n215 = local read "DataC1"() -> (w340:string[])
                        n216 = control-ref of="TableType"() -> (w322:refnum<vi>)
                        n217 = Build Array(w340, w320, w337) -> (w339:string[][])
                        n218 = local write "DataC2"(w320) -> ()
                        n219 = local write "DataC3"(w337) -> ()
                        n220 = Transpose 2D Array(2D array=w339) -> (transposed array=w338:string[][])
                        n221 = Strip Path(path=w327) -> (stripped path=w325:path, name=w329:string)
                        n222 = invoke class="CmbBox" method="Reinit To Default"(reference=w322) -> (error out=w323:errorcluster)  [unwired: 2 in, 2 out]
                        n223 = Index Array(array=w320, index=0) -> (element=w332:string)
                        n224 = local write "Folder Table"(w338) -> ()
                        n225 = Path To String(path=w325) -> (string=w330:string)
                        n226 = Empty String/Path?(string/path=w332) -> (empty?=w334:bool)
                        n227 = Build Array(w330, w329) -> (w328:string[])
                        n228 = Select(t=u32 16764057, s=w334, f=u32 5898138) -> (s? t:f=w326:u32)
                        n229 = property on="Folder Table" class="Tbl (strict)"("Active Cell"=T2 {"Row"=-1, "Column"=2} ("Active Cell:Active Cell"), "Cell BG Color"=u32 16448250, "Index Values"=T3 {"Row"=0, "Column"=0}) -> ()  [unwired: 2 in, 2 out]
                        n230 = property on="Folder Table" class="Tbl (strict)"("Column Headers[]"=w328, "Active Cell"=T2 {"Row"=-1, "Column"=1} ("Active Cell:Active Cell"), "Cell BG Color"=w326) -> ()  [unwired: 2 in, 2 out]
                        n231 = property on="TableType" class="CmbBox"(error in=w323, "Text.TextColor"=u32 16860) -> ()  [unwired: 1 in, 2 out]
                      }
                    }
                    n232 = stacked-sequence {
                      seq-local: [w348 _] -> [_ w351]
                      tunnel: w319 -> [w348 _]
                      frame #0 {
                        n233 = local read "PosC1"() -> (w350:T2)
                        n234 = property on="Folder Table" class="Tbl (strict)"("Active Cell"=w350, "Cell BG Color"=u32 16448250) -> ()  [unwired: 2 in, 2 out]
                        n235 = local read "PosC2"() -> (w347:T2)
                        n236 = property on="Folder Table" class="Tbl (strict)"("Active Cell"=w347, "Cell BG Color"=u32 16448250) -> ()  [unwired: 2 in, 2 out]
                        n237 = local read "PosC3"() -> (w345:T2)
                        n238 = property on="Folder Table" class="Tbl (strict)"("Active Cell"=w345, "Cell BG Color"=u32 16448250) -> ()  [unwired: 2 in, 2 out]
                      }
                      frame #1 {
                        n239 = property on="Folder Table" class="Tbl (strict)"("Active Cell"=w351, "Cell BG Color"=u32 16776817) -> ()  [unwired: 2 in, 2 out]
                        n240 = local write "PosC1"(w351) -> ()
                      }
                    }
                  }
                  frame 1 {
                    n241 = local read "DataC2"() -> (w356:string[])
                    n242 = local read "PathC1"() -> (w359:path)
                    n243 = Index Array(array=w356, index=w355) -> (element=w360:string)
                    n244 = Build Path(base path=w359, name or relative path=w360) -> (appended path=w358:path)
                    "PathC2" <- w358
                    n245 = call <vilib>:"Check if File or Folder Exists.vi"("path"=w358) -> ("file or folder exists?"=w353:bool, "dup path"=w357:path)  [unwired: 8 in, 1 out]
                    n246 = stacked-sequence {
                      seq-local: [w436 _] -> [_ w440]
                      tunnel: w361 -> [w436 _]
                      tunnel: [_ w439] -> w354
                      frame #0 {
                        n247 = local read "PosC2"() -> (w438:T2)
                        n248 = property on="Folder Table" class="Tbl (strict)"("Active Cell"=w438, "Cell BG Color"=u32 16448250) -> ()  [unwired: 2 in, 2 out]
                        n249 = local read "PosC3"() -> (w435:T2)
                        n250 = property on="Folder Table" class="Tbl (strict)"("Active Cell"=w435, "Cell BG Color"=u32 16448250) -> ()  [unwired: 2 in, 2 out]
                      }
                      frame #1 {
                        n251 = property on="Folder Table" class="Tbl (strict)"("Active Cell"=w440, "Cell BG Color"=u32 16776817) -> (error out=w439:errorcluster)  [unwired: 2 in, 1 out]
                        n252 = local write "PosC2"(w440) -> ()
                      }
                    }
                    n253 = case shown="True" w353 {
                      tunnel: w357 -> [_ w394]
                      tunnel: w354 -> [_ _]
                      frame False {
                      }
                      frame True {
                        n254 = local read "TableType"() -> (w374:string)
                        n255 = List Folder(path=w394) -> (path out=w381:path, folder names=w373:string[])  [unwired: 3 in, 2 out]
                        n256 = control-ref of="TableType"() -> (w364:refnum<vi>)
                        n257 = case shown="\"NG ONLY\"" w374 {
                          tunnel: [w397 w401 w419] -> w372
                          tunnel: w373 -> [w397 w400 w418]
                          tunnel: ["VIEW ALL" "OK ONLY" "NG ONLY"] -> w371
                          tunnel: [u32 16860 u32 40713 u32 16711680] -> w366
                          frame "VIEW ALL", Default {
                          }
                          frame "OK ONLY" {
                            n258 = for {
                              shift-right: [w410] -> w401
                              shift-left: string[] [] -> [w411]
                              tunnel: w400 -> [w409] mode=indexing
                              n259 = String Length(string=w409) -> (length=w404:i32)
                              n260 = Decrement(x=w404) -> (x-1=w403:i32)
                              n261 = String Subset(string=w409, offset (0)=w403, length (rest)=1 ("length (rest)")) -> (substring=w407:string)
                              n262 = Not Equal?(x=w407, y="!") -> (x != y?=w405:bool)
                              n263 = case shown="True" w405 {
                                tunnel: w411 -> [w412 w415]
                                tunnel: [w412 w414] -> w410
                                tunnel: w409 -> [_ w413]
                                frame False {
                                }
                                frame True {
                                n264 = Insert Into Array(array=w415, new element=w413) -> (w414:string[])  [unwired: 1 in]
                                }
                              }
                            }
                          }
                          frame "NG ONLY" {
                            n265 = for {
                              shift-right: [w428] -> w419
                              shift-left: string[] [] -> [w429]
                              tunnel: w418 -> [w423] mode=indexing
                              n266 = String Length(string=w423) -> (length=w422:i32)
                              n267 = Decrement(x=w422) -> (x-1=w421:i32)
                              n268 = String Subset(string=w423, offset (0)=w421, length (rest)=1 ("length (rest)")) -> (substring=w427:string)
                              n269 = Equal?(x=w427, y="!") -> (x = y?=w424:bool)
                              n270 = case shown="True" w424 {
                                tunnel: w429 -> [w430 w433]
                                tunnel: [w430 w432] -> w428
                                tunnel: w423 -> [_ w431]
                                frame False {
                                }
                                frame True {
                                n271 = Insert Into Array(array=w433, new element=w431) -> (w432:string[])  [unwired: 1 in]
                                }
                              }
                            }
                          }
                        }
                        n272 = invoke class="CmbBox" method="Reinit To Default"(reference=w364) -> (error out=w365:errorcluster)  [unwired: 2 in, 2 out]
                        n273 = local read "MasterPath"() -> (w378:path)
                        n274 = property on="TableType" class="CmbBox"(error in=w365, "Text.TextColor"=u32 16860) -> ()  [unwired: 1 in, 2 out]
                        n275 = Strip Path(path=w381) -> (stripped path=w380:path, name=w376:string)
                        n276 = Path To String(path=w378) -> (string=w384:string)
                        n277 = Strip Path(path=w380) -> (name=w377:string)  [unwired: 1 out]
                        n278 = Array Size(array=w372) -> (size(s)=w362:i32)
                        n279 = Index Array(array=w372, index=0) -> (element=w386:string)
                        n280 = local read "DataC1"() -> (w393:string[])
                        n281 = local read "DataC2"() -> (w382:string[])
                        n282 = Number To Decimal String(number=w362) -> (decimal integer string=w369:string)  [unwired: 1 in]
                        "FileCount" <- w369
                        n283 = Empty String/Path?(string/path=w386) -> (empty?=w388:bool)
                        n284 = Build Array(w384, w377, w376) -> (w379:string[])
                        n285 = Select(t=u32 16764057, s=w388, f=u32 5898138) -> (s? t:f=w383:u32)
                        n286 = Build Array(w393, w382, w372) -> (w392:string[][])
                        n287 = Concatenate Strings(w371, " (" ("string"), w369, ")" ("decimal integer string")) -> (w367:string)
                        n288 = Transpose 2D Array(2D array=w392) -> (transposed array=w391:string[][])
                        n289 = local write "Folder Table"(w391) -> ()
                        n290 = property on="TableType" class="CmbBox"("Val(Sgnl)"=w367, "Text.TextColor"=w366) -> ()  [unwired: 2 in, 2 out]
                        n291 = property on="Folder Table" class="Tbl (strict)"("Column Headers[]"=w379, "Active Cell"=T2 {"Row"=-1, "Column"=2} ("Active Cell:Active Cell"), "Cell BG Color"=w383, "Index Values"=T3 {"Row"=0, "Column"=0}) -> ()  [unwired: 2 in, 2 out]
                        n292 = local write "DataC3"(w372) -> ()
                      }
                    }
                  }
                  frame 2 {
                    n293 = local read "DataC3"() -> (w453:string[])
                    n294 = local read "PathC2"() -> (w457:path)
                    n295 = Unbundle By Name(w451) -> ("Row"=w450:i32)
                    n296 = Index Array(array=w453, index=w452) -> (element=w458:string)
                    n297 = Subtract(x=w450, y=10) -> (x-y=w443:i32)
                    n298 = Build Path(base path=w457, name or relative path=w458) -> (appended path=w456:path)
                    "PathC3" <- w456
                    n299 = Less Than 0?(x=w443) -> (x < 0?=w448:bool)
                    n300 = Select(t=0 ("y"), s=w448, f=w443) -> (s? t:f=w445:i32)
                    n301 = call <vilib>:"Check if File or Folder Exists.vi"("path"=w456) -> ("file or folder exists?"=w455:bool, "dup path"=w454:path)  [unwired: 8 in, 1 out]
                    n302 = Bundle By Name(cluster=T3 {"Row"=0, "Column"=0} ("Index Values"), "Column"=u32 0, "Row"=w445) -> (w447:T3)
                    n303 = case shown="True" w455 {
                      tunnel: w454 -> [_ w470]
                      tunnel: w447 -> [_ w468]
                      frame False {
                      }
                      frame True {
                        n304 = property on="Folder Table" class="Tbl (strict)"("Index Values"=w468) -> ()  [unwired: 2 in, 2 out]
                        n305 = local write "Display"(TRUE ("Display")) -> ()
                        n306 = List Folder(path=w470) -> (path out=w467:path, filenames=w464:string[])  [unwired: 3 in, 2 out]
                        "DataC4" <- w464
                        n307 = for {
                          tunnel: w464 -> [w471] mode=indexing
                          tunnel: "_Result.csv" ("regular expression") -> [w474]
                          tunnel: [w471] -> w465
                          stop <- w473 stop-if-true
                          n308 = String Subset(string=w471, offset (0)=4) -> (substring=w472:string)  [unwired: 1 in]
                          n309 = Equal?(x=w472, y=w474) -> (x = y?=w473:bool)
                        }
                        n310 = Build Path(base path=w467, name or relative path=w465) -> (appended path=w459:path)
                        n311 = call-poly <vilib>:"Read Delimited Spreadsheet.vi"("file path (dialog if empty)"=w459, "transpose? (F)"=FALSE, "delimiter (\\t)"="," ("delimiter (\\t)")) -> ("all rows"=→"ResultTest":string[][], "error out"=w460:errorcluster)  [unwired: 7 in, 4 out]
                        n312 = call <vilib>:"Clear Errors.vi"("error in (no error)"=w460) -> ()  [unwired: 5 in, 2 out]
                      }
                    }
                    n313 = stacked-sequence {
                      seq-local: [w476 _] -> [_ w479]
                      tunnel: w451 -> [w476 _]
                      frame #0 {
                        n314 = local read "PosC3"() -> (w478:T2)
                        n315 = property on="Folder Table" class="Tbl (strict)"("Active Cell"=w478, "Cell BG Color"=u32 16448250) -> ()  [unwired: 2 in, 2 out]
                      }
                      frame #1 {
                        n316 = property on="Folder Table" class="Tbl (strict)"("Active Cell"=w479, "Cell BG Color"=u32 16776817) -> ()  [unwired: 2 in, 2 out]
                        n317 = local write "PosC3"(w479) -> ()
                      }
                    }
                  }
                }
              }
            }
          }
          event "TableType": Value Change {
            n318 = event-data() -> ()  [unwired: 1 in, 6 out]
            n319 = local read "PosC3"() -> (w497:T2)
            n320 = local read "PosC2"() -> (w484:T2)
            n321 = local read "DataC2"() -> (w495:string[])
            n322 = local read "PathC2"() -> (w494:path)
            n323 = local read "TableType"() -> (w492:string)
            n324 = List Folder(path=w494) -> (path out=w491:path, folder names=w493:string[])  [unwired: 3 in, 2 out]
            n325 = property on="Folder Table" class="Tbl (strict)"("Active Cell"=w497, "Cell BG Color"=u32 16777225) -> ()  [unwired: 2 in, 2 out]
            n326 = case shown="\"NG ONLY\"" w492 {
              tunnel: [w527 w531 w549] -> w483
              tunnel: w493 -> [w527 w530 w548]
              tunnel: ["VIEW ALL" "OK ONLY" "NG ONLY"] -> w482
              tunnel: [u32 16860 u32 40713 u32 16711680] -> w481
              frame "VIEW ALL", Default {
              }
              frame "OK ONLY" {
                n327 = for {
                  shift-right: [w540] -> w531
                  shift-left: string[] [] -> [w541]
                  tunnel: w530 -> [w536] mode=indexing
                  n328 = String Length(string=w536) -> (length=w533:i32)
                  n329 = Decrement(x=w533) -> (x-1=w534:i32)
                  n330 = String Subset(string=w536, offset (0)=w534, length (rest)=1 ("length (rest)")) -> (substring=w539:string)
                  n331 = Not Equal?(x=w539, y="!") -> (x != y?=w535:bool)
                  n332 = case shown="True" w535 {
                    tunnel: w541 -> [w542 w545]
                    tunnel: [w542 w544] -> w540
                    tunnel: w536 -> [_ w543]
                    frame False {
                    }
                    frame True {
                      n333 = Insert Into Array(array=w545, new element=w543) -> (w544:string[])  [unwired: 1 in]
                    }
                  }
                }
              }
              frame "NG ONLY" {
                n334 = for {
                  shift-right: [w558] -> w549
                  shift-left: string[] [] -> [w559]
                  tunnel: w548 -> [w554] mode=indexing
                  n335 = String Length(string=w554) -> (length=w551:i32)
                  n336 = Decrement(x=w551) -> (x-1=w552:i32)
                  n337 = String Subset(string=w554, offset (0)=w552, length (rest)=1 ("length (rest)")) -> (substring=w557:string)
                  n338 = Equal?(x=w557, y="!") -> (x = y?=w553:bool)
                  n339 = case shown="True" w553 {
                    tunnel: w559 -> [w560 w563]
                    tunnel: [w560 w562] -> w558
                    tunnel: w554 -> [_ w561]
                    frame False {
                    }
                    frame True {
                      n340 = Insert Into Array(array=w563, new element=w561) -> (w562:string[])  [unwired: 1 in]
                    }
                  }
                }
              }
            }
            n341 = Empty Array?(array=w495) -> (empty?=w487:bool)
            n342 = Unbundle By Name(w484) -> ("Column"=w490:i32)
            n343 = Equal?(x=w490, y=1) -> (x = y?=w486:bool)
            n344 = Not(x=w487) -> (.not. x?=w485:bool)
            n345 = And(x=w486, y=w485) -> (x .and. y?=w488:bool)
            n346 = case shown="True" w488 {
              tunnel: w483 -> [_ w500]
              tunnel: w491 -> [_ w506]
              tunnel: w482 -> [_ w499]
              tunnel: w481 -> [_ w498]
              frame False {
              }
              frame True {
                n347 = local read "MasterPath"() -> (w522:path)
                n348 = Strip Path(path=w506) -> (stripped path=w520:path, name=w524:string)
                n349 = Path To String(path=w522) -> (string=w517:string)
                n350 = Strip Path(path=w520) -> (name=w523:string)  [unwired: 1 out]
                n351 = Index Array(array=w500, index=0) -> (element=w516:string)
                n352 = local read "DataC1"() -> (w512:string[])
                n353 = local read "DataC2"() -> (w519:string[])
                n354 = Array Size(array=w500) -> (size(s)=w505:i32)
                n355 = Number To Decimal String(number=w505) -> (decimal integer string=w504:string)  [unwired: 1 in]
                n356 = Empty String/Path?(string/path=w516) -> (empty?=w515:bool)
                n357 = Build Array(w517, w523, w524) -> (w521:string[])
                n358 = Select(t=u32 16764057, s=w515, f=u32 5898138) -> (s? t:f=w518:u32)
                n359 = Build Array(w512, w519, w500) -> (w513:string[][])
                n360 = Transpose 2D Array(2D array=w513) -> (transposed array=w514:string[][])
                n361 = Concatenate Strings(w499, " (" ("string"), w504, ")" ("decimal integer string")) -> (w503:string)
                n362 = local write "Folder Table"(w514) -> ()
                n363 = property on="TableType" class="CmbBox"("Value"=w503, "Text.TextColor"=w498) -> ()  [unwired: 2 in, 2 out]
                n364 = property on="Folder Table" class="Tbl (strict)"("Column Headers[]"=w521, "Active Cell"=T2 {"Row"=-1, "Column"=2} ("Active Cell:Active Cell"), "Cell BG Color"=w518, "Index Values"=T3 {"Row"=0, "Column"=0}) -> ()  [unwired: 2 in, 2 out]
                n365 = local write "DataC3"(w500) -> ()
              }
            }
          }
        }
        n366 = disable-structure shown="Enabled" {
          frame Enabled {
            n367 = local read "Display"() -> (w28:bool)
            n368 = case shown="True" w28 {
              frame False {
              }
              frame True {
                n369 = stacked-sequence {
                  frame #0 {
                    n370 = local read "ResultTest"() -> (w97:string[][])
                    n371 = local write "Display"(FALSE ("Disp2")) -> ()
                    n372 = Index Array(array=w97, index (col)=1 ("disabled index (col)")) -> (element=w95:string[])  [unwired: 1 in]
                    n373 = Split 1D Array(array=w95, index=3) -> (first subarray=w93:string[], second subarray=w89:string[])
                    "ResultGraph" <- w89
                    n374 = Index Array(array=w93) -> (element #1=→"PRODUCT No.":string, element #2=→"LANE  No.":string, element #3=→"LASER  No.":string)  [unwired: 3 in]
                    n375 = for {
                      tunnel: w89 -> [w102] mode=indexing
                      tunnel: [w101] -> w90 mode=indexing
                      n376 = case shown="\"4\"" w102 {
                        tunnel: [u32 12124152 u32 1891328 u32 16740734] -> w101
                        frame "0", Default {
                        }
                        frame "1" {
                        }
                        frame "4" {
                        }
                      }
                    }
                    n377 = Index Array(array=w89, index=27) -> (element=w87:string)
                    n378 = Index Array(array=w90) -> (element #1=w58:u32, element #2=w59:u32, element #3=w60:u32, element #4=w61:u32, element #5=w62:u32, element #6=w63:u32, element #7=w64:u32, element #8=w65:u32, element #9=w66:u32, element #10=w67:u32, element #11=w68:u32, element #12=w69:u32, element #13=w70:u32, element #14=w71:u32, element #15=w72:u32, element #16=w73:u32, element #17=w74:u32, element #18=w75:u32, element #19=w76:u32, element #20=w77:u32, element #21=w78:u32, element #22=w79:u32, element #23=w80:u32, element #24=w81:u32, element #25=w82:u32, element #26=w83:u32, element #27=w84:u32, element #28=w30:u32)  [unwired: 28 in]
                    n379 = case shown="\"4\"" w87 {
                      tunnel: ["NC" "OK" "NG"] -> w29
                      frame "0", Default {
                      }
                      frame "1" {
                      }
                      frame "4" {
                      }
                    }
                    "RESULT" <- w29
                    n380 = property on="Megga Test" class="Str"("Text.BGColor"=w58) -> ()  [unwired: 2 in, 2 out]
                    n381 = property on="WDW Locked" class="Str"("Text.BGColor"=w59) -> ()  [unwired: 2 in, 2 out]
                    n382 = property on="WDW Unlocked" class="Str"("Text.BGColor"=w60) -> ()  [unwired: 2 in, 2 out]
                    n383 = property on="Door Lock" class="Str"("Text.BGColor"=w61) -> ()  [unwired: 2 in, 2 out]
                    n384 = property on="Door Unlocked" class="Str"("Text.BGColor"=w62) -> ()  [unwired: 2 in, 2 out]
                    n385 = property on="FR Man Up" class="Str"("Text.BGColor"=w63) -> ()  [unwired: 2 in, 2 out]
                    n386 = property on="FR Man Down" class="Str"("Text.BGColor"=w64) -> ()  [unwired: 2 in, 2 out]
                    n387 = property on="FR Auto Up" class="Str"("Text.BGColor"=w65) -> ()  [unwired: 2 in, 2 out]
                    n388 = property on="FR Auto Down" class="Str"("Text.BGColor"=w66) -> ()  [unwired: 2 in, 2 out]
                    n389 = property on="RR Man Up" class="Str"("Text.BGColor"=w67) -> ()  [unwired: 2 in, 2 out]
                    n390 = property on="RR Man Down" class="Str"("Text.BGColor"=w68) -> ()  [unwired: 2 in, 2 out]
                    n391 = property on="FL Man Up" class="Str"("Text.BGColor"=w69) -> ()  [unwired: 2 in, 2 out]
                    n392 = property on="FL Man Down" class="Str"("Text.BGColor"=w70) -> ()  [unwired: 2 in, 2 out]
                    n393 = property on="FL Auto Up" class="Str"("Text.BGColor"=w71) -> ()  [unwired: 2 in, 2 out]
                    n394 = property on="FL Auto Down" class="Str"("Text.BGColor"=w72) -> ()  [unwired: 2 in, 2 out]
                    n395 = property on="RL Man Up" class="Str"("Text.BGColor"=w73) -> ()  [unwired: 2 in, 2 out]
                    n396 = property on="RL Man Down" class="Str"("Text.BGColor"=w74) -> ()  [unwired: 2 in, 2 out]
                    n397 = property on="LIN DR Up" class="Str"("Text.BGColor"=w75) -> ()  [unwired: 2 in, 2 out]
                    n398 = property on="LIN DR Down" class="Str"("Text.BGColor"=w76) -> ()  [unwired: 2 in, 2 out]
                    n399 = property on="LIN DR Auto" class="Str"("Text.BGColor"=w77) -> ()  [unwired: 2 in, 2 out]
                    n400 = property on="LIN AS Up" class="Str"("Text.BGColor"=w78) -> ()  [unwired: 2 in, 2 out]
                    n401 = property on="LIN AS Down" class="Str"("Text.BGColor"=w79) -> ()  [unwired: 2 in, 2 out]
                    n402 = property on="LIN AS Auto" class="Str"("Text.BGColor"=w80) -> ()  [unwired: 2 in, 2 out]
                    n403 = property on="LIN WDW Lock" class="Str"("Text.BGColor"=w81) -> ()  [unwired: 2 in, 2 out]
                    n404 = property on="Vision Pad" class="Str"("Text.BGColor"=w82) -> ()  [unwired: 2 in, 2 out]
                    n405 = property on="Vision Pin" class="Str"("Text.BGColor"=w83) -> ()  [unwired: 2 in, 2 out]
                    n406 = property on="QR Code" class="Str"("Text.BGColor"=w84) -> ()  [unwired: 2 in, 2 out]
                    n407 = property on="RESULT" class="Str"("Text.BGColor"=w30) -> ()  [unwired: 2 in, 2 out]
                    "Megga Test" <- "Mega Test" ("Megga Test")
                    "WDW Locked" <- "WDW Locked" ("Megga Test")
                    "WDW Unlocked" <- "WDW Unlocked" ("Megga Test")
                    "Door Lock" <- "Door Locked" ("Megga Test")
                    "Door Unlocked" <- "Door Unlocked" ("Megga Test")
                    "FR Man Up" <- "FR Man Up" ("Megga Test")
                    "FR Man Down" <- "FR Man Down" ("Megga Test")
                    "FR Auto Up" <- "FR Auto Up" ("Megga Test")
                    "FR Auto Down" <- "FR Auto Down" ("Megga Test")
                    "RR Man Up" <- "RR Man Up" ("Megga Test")
                    "RR Man Down" <- "RR Man Down" ("Megga Test")
                    "FL Man Up" <- "FL Man Up" ("Megga Test")
                    "FL Man Down" <- "FL Man Down" ("Megga Test")
                    "FL Auto Up" <- "FL Auto Up" ("Megga Test")
                    "FL Auto Down" <- "FL Auto Down" ("Megga Test")
                    "RL Man Up" <- "RL Man Up" ("Megga Test")
                    "RL Man Down" <- "RL Man Down" ("Megga Test")
                    "LIN DR Up" <- "LIN DR Up" ("Megga Test")
                    "LIN DR Down" <- "LIN DR Down" ("Megga Test")
                    "LIN DR Auto" <- "LIN DR Auto" ("Megga Test")
                    "LIN AS Up" <- "LIN AS Up" ("Megga Test")
                    "LIN AS Down" <- "LIN AS Down" ("Megga Test")
                    "LIN AS Auto" <- "LIN AS Auto" ("Megga Test")
                    "LIN WDW Lock" <- "LIN WDW Lock" ("Megga Test")
                    "Vision Pad" <- "Vision ILLU." ("Megga Test")
                    "Vision Pin" <- "Vision Pin" ("Megga Test")
                    "QR Code" <- "QR Code" ("Megga Test")
                  }
                  frame #1 {
                    w106 = sgl 1.2 ("Zoom Factor")
                    n408 = local read "PathC3"() -> (w120:path)
                    n409 = local read "DataC4"() -> (w121:string[])
                    n410 = call "FilterBMP.vi"("Filenames"=w121, "Path"=w120) -> ("BMP Path"=w119:path[])  [unwired: 8 in, 1 out]
                    n411 = Index Array(array=w119) -> (element #1=w118:path, element #2=w117:path, element #3=w116:path, element #4=w115:path, element #5=w114:path, element #6=w113:path, element #7=w112:path, element #8=w111:path, element #9=w110:path, element #10=w109:path, element #11=w108:path, element #12=w107:path)  [unwired: 12 in]
                    n412 = call "ShowBMP.vi"("PathBMP_Up"=w117, "PathBMP_Down"=w118) -> ("Image_Up"=→"WDWG_Unlock":picture, "Image_Down"=→"WDWG_Lock":picture)  [unwired: 8 in]
                    n413 = call "ShowBMP.vi"("PathBMP_Up"=w115, "PathBMP_Down"=w116) -> ("Image_Up"=→"DLG_Unlock":picture, "Image_Down"=→"DLG_Lock":picture)  [unwired: 8 in]
                    n414 = call "ShowBMP.vi"("PathBMP_Up"=w113, "PathBMP_Down"=w114) -> ("Image_Up"=→"FRG_Up":picture, "Image_Down"=→"FRG_Down":picture)  [unwired: 8 in]
                    n415 = call "ShowBMP.vi"("PathBMP_Up"=w111, "PathBMP_Down"=w112) -> ("Image_Up"=→"RRG_Up":picture, "Image_Down"=→"RRG_Down":picture)  [unwired: 8 in]
                    n416 = call "ShowBMP.vi"("PathBMP_Up"=w109, "PathBMP_Down"=w110) -> ("Image_Up"=→"FLG_Up":picture, "Image_Down"=→"FLG_Down":picture)  [unwired: 8 in]
                    n417 = call "ShowBMP.vi"("PathBMP_Up"=w107, "PathBMP_Down"=w108) -> ("Image_Up"=→"RLG_Up":picture, "Image_Down"=→"RLG_Down":picture)  [unwired: 8 in]
                    n418 = property on="WDWG_Lock" class="Pict"("ZoomFactor"=w106) -> ()  [unwired: 2 in, 2 out]
                    n419 = property on="WDWG_Unlock" class="Pict"("ZoomFactor"=w106) -> ()  [unwired: 2 in, 2 out]
                    n420 = property on="DLG_Lock" class="Pict"("ZoomFactor"=w106) -> ()  [unwired: 2 in, 2 out]
                    n421 = property on="DLG_Unlock" class="Pict"("ZoomFactor"=w106) -> ()  [unwired: 2 in, 2 out]
                    n422 = property on="FRG_Down" class="Pict"("ZoomFactor"=w106) -> ()  [unwired: 2 in, 2 out]
                    n423 = property on="FRG_Up" class="Pict"("ZoomFactor"=w106) -> ()  [unwired: 2 in, 2 out]
                    n424 = property on="RRG_Down" class="Pict"("ZoomFactor"=w106) -> ()  [unwired: 2 in, 2 out]
                    n425 = property on="RRG_Up" class="Pict"("ZoomFactor"=w106) -> ()  [unwired: 2 in, 2 out]
                    n426 = property on="FLG_Down" class="Pict"("ZoomFactor"=w106) -> ()  [unwired: 2 in, 2 out]
                    n427 = property on="FLG_Up" class="Pict"("ZoomFactor"=w106) -> ()  [unwired: 2 in, 2 out]
                    n428 = property on="RLG_Down" class="Pict"("ZoomFactor"=w106) -> ()  [unwired: 2 in, 2 out]
                    n429 = property on="RLG_Up" class="Pict"("ZoomFactor"=w106) -> ()  [unwired: 2 in, 2 out]
                  }
                }
              }
            }
          }
          frame Disabled {
          }
        }
      }
    }
  }
